vi "Do Turn.vi"(11 "Game in":refnum<class "Game.lvclass">) -> (3 "Game out":refnum<class "Game.lvclass">)   [LabVIEW 2020, in "SquareBattle.lvlib" / "Game.lvclass"]
uses:
  Game.lvclass
  Game.lvclass/Game.ctl
  Team/Team.lvclass/Team.ctl
  Team/Team.lvclass
  Map/Map.lvclass
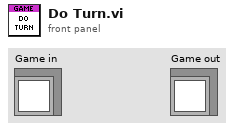
[diagram p1: front panel]
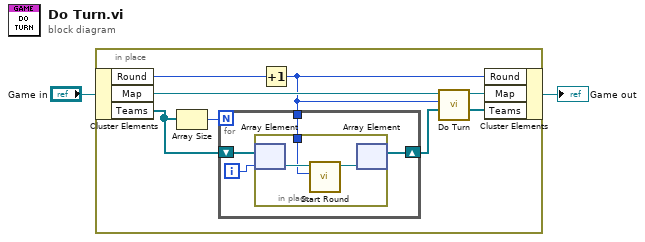
[diagram p0: block diagram]
diagram:
  n1 = in-place {
    n2 = in-place-cluster #1("Game in") -> ("Round"=w10:u32, "Map"=w9:refnum<class "Map.lvclass">, "Teams"=w6:refnum<class "Team.lvclass">[])
    n3 = Array Size(array=w6) -> (size(s)=w5:i32)
    n4 = Increment(x=w10) -> (x+1=w4:u32)
    n5 = for {
      N: w5 -> [_]
      shift-right: [w11] -> w3
      shift-left: w6 -> [w14]
      tunnel: w4 -> [w12]
      i -> [w13]
      n6 = in-place {
        in-place-border: w12 -> [w16]
        n7 = in-place-array #2(w14, w13) -> (w17:refnum<class "Team.lvclass">)
        n8 = call "Start Round.vi"("Round"=w16, "Team in"=w17) -> ("Team out"=w15:refnum<class "Team.lvclass">)  [unwired: 9 in]
        n9 = in-place-array #2(w15) -> (w11:refnum<class "Team.lvclass">[])  [unwired: 1 out]
      }
    }
    n10 = call "Do Turn.vi"("Teams In"=w3, "Round"=w4, "Map in"=w9) -> ("Teams"=w7:refnum<class "Team.lvclass">[], "Map out"=w8:refnum<class "Map.lvclass">)  [unwired: 7 in]
    n11 = in-place-cluster #1("Round"=w4, "Map"=w8, "Teams"=w7) -> (→"Game out":refnum<class "Game.lvclass">)
  }
